vi "Main Draft LIEF Imager.vi"() -> ()   [LabVIEW 2016]
uses:
  Imager Editor Handler/Imager Handler.lvclass
  C:/Program Files (x86)/National Instruments/LabVIEW 2016/vi.lib/LIEF/Image Editor Handler/Image Editor Handler.lvclass
  Imager Editor Handler/Imager Handler.lvclass/Imager Handler.ctl
  Imager Editor Handler/Write Properties Pane.vi
  Imager Editor Handler/Write SystemPropertyChanged Event.vi
  <vilib>/LIEF/Image Editor Handler/Image Editor Handler.lvclass
  <vilib>/nisyscfg/nisyscfg.lvlib
panel:
  in  "Search":bool
  in  "Collapse":bool caption="Last"
  in  "2D Picture":picture
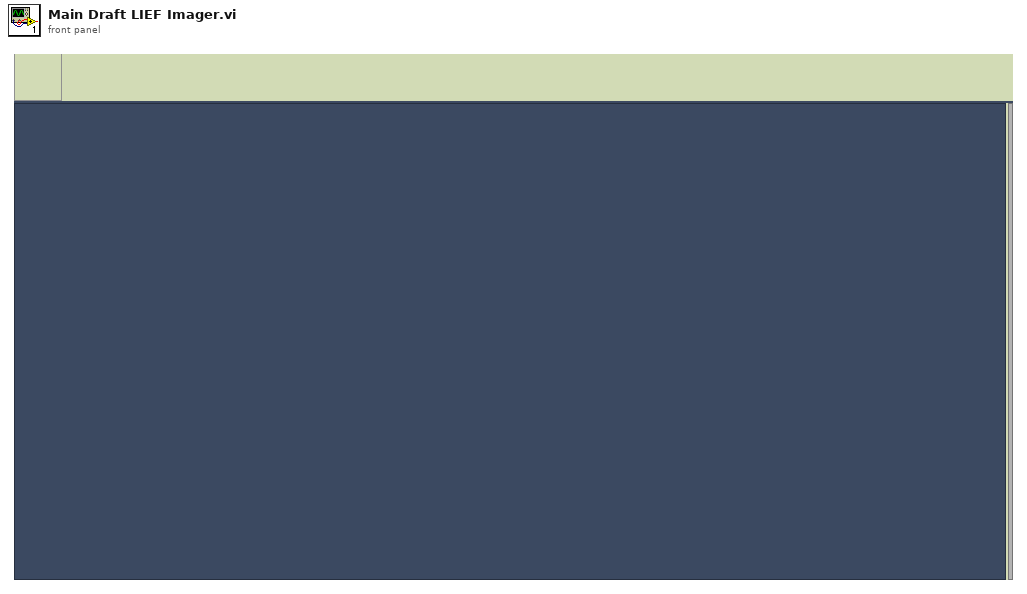
[diagram p1: front panel]
types:
  T1 = enum32{"invalid app kind", "Development System", "Run Time System", "Student Edition", "Embedded LabVIEW", "Evaluation", "Custom"}
  T2 = typedef "LVBoundsTypeDef.ctl" = cluster{"Width":u32, "Height":u32}
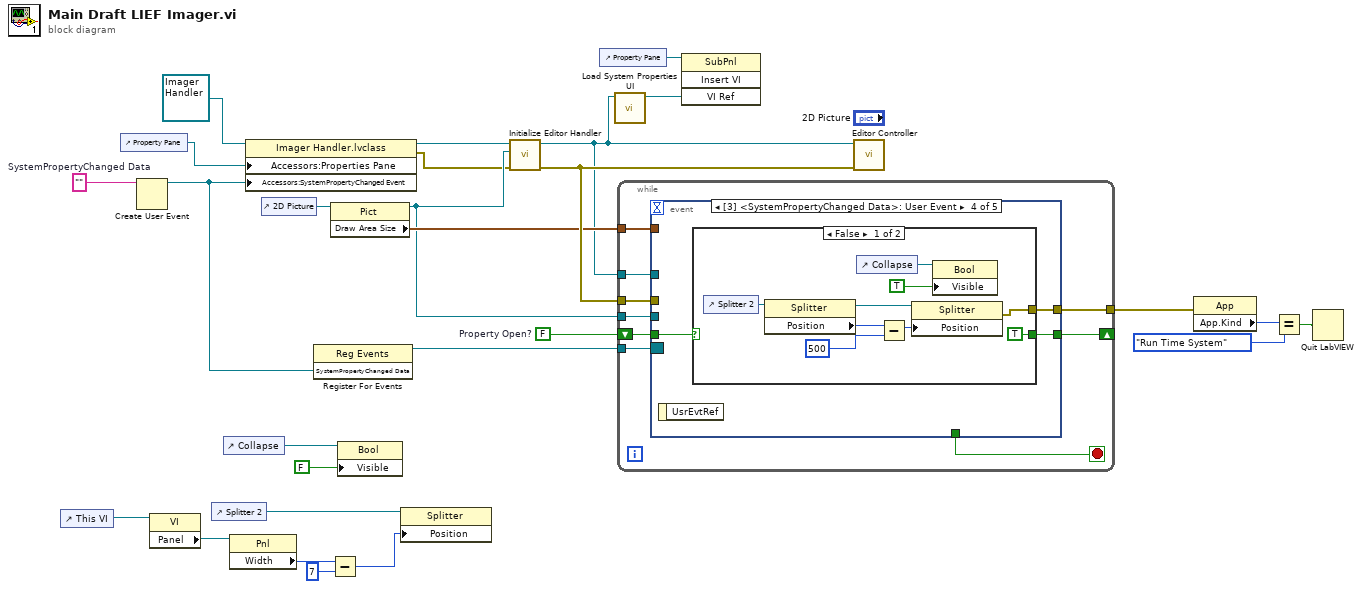
[diagram p0: block diagram]
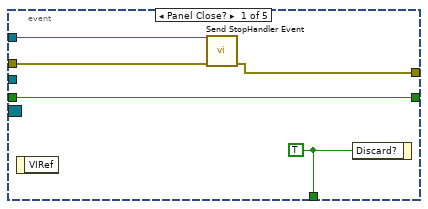
[diagram p2: hidden frame]
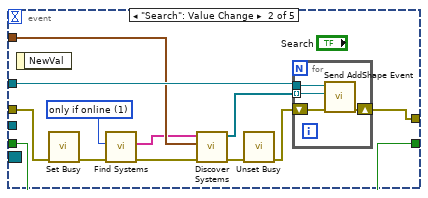
[diagram p3: hidden frame]
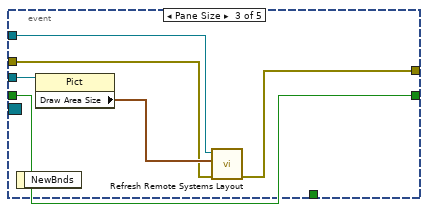
[diagram p4: hidden frame]
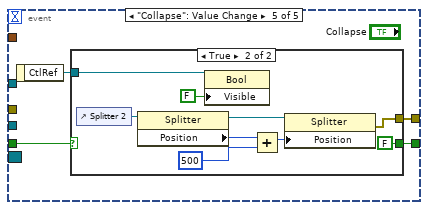
[diagram p6: hidden frame]
diagram:
  w15 = FALSE  # Property Open?
  w24 = ""  # SystemPropertyChanged Data
  n1 = control-ref of="This VI"() -> (w14:refnum<vi>)
  n2 = control-ref of="Property Pane"() -> (w18:refnum<vi>)
  n3 = Create User Event(user event datatype=w24) -> (user event=w20:refnum<user-event>)  [unwired: 1 in, 1 out]
  n4 = property class="VI"(reference=w14) -> ("Panel"=w13:refnum<vi>)  [unwired: 1 in, 2 out]
  n5 = control-ref of="Splitter 2"() -> (w12:refnum<vi>)
  n6 = control-ref of="Collapse"() -> (w17:refnum<vi>)
  n7 = property class="Pnl"(reference=w13) -> ("Width"=w11:u32)  [unwired: 1 in, 2 out]
  n8 = property class="Imager Handler.lvclass"(reference=refnum<class "Imager Handler.lvclass"> refnum ("Imager Handler.lvclass"), "Accessors:Properties Pane"=w18, "Accessors:SystemPropertyChanged Event"=w20) -> (reference out=w22:refnum<class "Imager Handler.lvclass">, error out=w5:errorcluster)  [unwired: 1 in]
  n9 = control-ref of="2D Picture"() -> (w27:refnum<vi>)
  n10 = register-events(w20) -> (reference out=w19:refnum<event-registration>)  [unwired: 2 in, 1 out]
  n11 = Subtract(x=w11, y=u32 7) -> (x-y=w9:u32)
  n12 = property class="Pict"(reference=w27) -> (reference out=w21:refnum<vi>, "Draw Area Size"=w25:T2)  [unwired: 1 in, 1 out]
  n13 = property class="Bool"(reference=w17, "Visible"=FALSE) -> ()  [unwired: 1 in, 2 out]
  n14 = property class="Splitter"(reference=w12, "Position"=w9) -> ()  [unwired: 1 in, 2 out]
  n15 = call <vilib>:"Initialize Editor Handler.vi"("error in (no error)"=w5, "PictureRef"=w21, "Editor Handler in"=w22) -> ("error out"=w26:errorcluster, "Editor Handler out"=w6:refnum<class "Imager Handler.lvclass">)  [unwired: 7 in]
  n16 = control-ref of="Property Pane"() -> (w8:refnum<vi>)
  n17 = call "Load System Properties UI.vi"("Editor Handler out"=w6) -> ("VI out"=w7:refnum<vi>)  [unwired: 9 in, 1 out]
  n18 = while {
    tunnel: w6 -> [w35]
    tunnel: w26 -> [w34]
    tunnel: w25 -> [w33]
    tunnel: w21 -> [w32]
    tunnel: w19 -> [w31]
    shift-right: [w29] -> _
    shift-left: w15 -> [w30]
    tunnel: [w28] -> w1
    stop <- w36 stop-if-true
    n19 = event shown="[3] <SystemPropertyChanged Data>: User Event" {
      selector: w31 -> [_ _ _ _ _]
      dyn-events: _ -> [_ _ _ _ _]
      timeout: _ -> [_ _ _ _ _]
      tunnel: [w41 _ _ _ _] -> w36
      tunnel: w35 -> [w40 w51 w59 _ _]
      tunnel: w34 -> [w39 w53 w61 _ _]
      tunnel: w33 -> [_ w50 _ _ _]
      tunnel: w32 -> [_ _ w63 _ _]
      tunnel: w30 -> [w38 w43 w60 w66 w79]
      tunnel: [w38 w43 w60 w65 w78] -> w29
      tunnel: [w37 w42 w58 w64 w77] -> w28
      event Panel Close? {
        w41 = TRUE ("Discard?")
        n20 = event-data() -> ()  [unwired: 1 in, 1 out]
        n21 = call <vilib>:"Send StopHandler Event.vi"("error in (no error)"=w39, "Editor Handler in"=w40) -> ("error out"=w37:errorcluster)  [unwired: 8 in, 1 out]
        n22 = event-data("Discard?"=w41) -> ()  [unwired: 1 in, 1 out]
      }
      event "Search": Value Change {
        w48 = u32 1 items=["none"=0, "only if online"=1, "all"=3] ("Include Cached Results (all)")
        n23 = event-data() -> ()  [unwired: 1 in, 1 out]
        n24 = call <vilib>:"Set Busy.vi"("error in (no error)"=w53) -> ("error out"=w47:errorcluster)  [unwired: 9 in, 1 out]
        n25 = call <vilib>:"Find Systems.vi"("error in (no error)"=w47, "Include Cached Results (all)"=w48) -> ("error out"=w46:errorcluster, "Detected Systems"=w45:string[])  [unwired: 7 in, 1 out]
        n26 = call "Discover Systems.vi"("error in (no error)"=w46, "Draw Area Size"=w50, "Detected Systems"=w45) -> ("error out"=w52:errorcluster, "RemoteSys Found"=w44:refnum<data-value>[])  [unwired: 5 in, 2 out]
        n27 = call <vilib>:"Unset Busy.vi"("error in (no error)"=w52) -> ("error out"=w49:errorcluster)  [unwired: 10 in]
        n28 = for {
          tunnel: w51 -> [w57]
          tunnel: w44 -> [w56] mode=indexing
          shift-right: [w54] -> w42
          shift-left: w49 -> [w55]
          n29 = call <vilib>:"Send AddShape Event.vi"("error in (no error)"=w55, "New Shape Reference"=w56, "Editor Handler in"=w57) -> ("error out"=w54:errorcluster)  [unwired: 7 in, 1 out]
        }
      }
      event Pane Size {
        n30 = event-data() -> ()  [unwired: 1 in, 1 out]
        n31 = property class="Pict"(reference=w63) -> ("Draw Area Size"=w62:T2)  [unwired: 1 in, 2 out]
        n32 = call "Refresh Remote Systems Layout.vi"("error in (no error)"=w61, "Draw Area Size"=w62, "Editor Handler in"=w59) -> ("error out"=w58:errorcluster)  [unwired: 8 in]
      }
      event User Event {
        n33 = event-data() -> ()  [unwired: 1 in, 1 out]
        n34 = case shown="False" w66 {
          selector: w66 -> [_ w76]
          tunnel: [TRUE ("Visible") w76] -> w65
          tunnel: [w67 _] -> w64
          frame False {
            n35 = control-ref of="Splitter 2"() -> (w75:refnum<vi>)
            n36 = property class="Splitter"(reference=w75) -> (reference out=w72:refnum<vi>, "Position"=w74:i32)  [unwired: 1 in, 1 out]
            n37 = control-ref of="Collapse"() -> (w70:refnum<vi>)
            n38 = Subtract(x=w74, y=500) -> (x-y=w71:i32)
            n39 = property class="Splitter"(reference=w72, "Position"=w71) -> (error out=w67:errorcluster)  [unwired: 1 in, 1 out]
            n40 = property class="Bool"(reference=w70, "Visible"=TRUE) -> ()  [unwired: 1 in, 2 out]
          }
          frame True {
          }
        }
      }
      event "Collapse": Value Change {
        n41 = event-data() -> ("CtlRef"=w80:refnum<vi>)  [unwired: 1 in]
        n42 = case shown="True" w79 {
          selector: w79 -> [w81 _]
          tunnel: w80 -> [_ w90]
          tunnel: [w81 FALSE ("Visible")] -> w78
          tunnel: [_ w82] -> w77
          frame False {
          }
          frame True {
            n43 = control-ref of="Splitter 2"() -> (w88:refnum<vi>)
            n44 = property class="Splitter"(reference=w88) -> (reference out=w85:refnum<vi>, "Position"=w87:i32)  [unwired: 1 in, 1 out]
            n45 = property class="Bool"(reference=w90, "Visible"=FALSE) -> ()  [unwired: 1 in, 2 out]
            n46 = Add(x=w87, y=500) -> (x+y=w84:i32)
            n47 = property class="Splitter"(reference=w85, "Position"=w84) -> (error out=w82:errorcluster)  [unwired: 1 in, 1 out]
          }
        }
      }
    }
  }
  n48 = invoke class="SubPnl" method="Insert VI"(reference=w8, "VI Ref"=w7) -> ()  [unwired: 2 in, 4 out]
  n49 = call <vilib>:"Editor Controller.vi"("error in (no error)"=w26, "Editor Handler in"=w6) -> ()  [unwired: 8 in, 2 out]
  n50 = property class="App"(error in=w1) -> ("App.Kind"=w4:T1)  [unwired: 1 in, 2 out]
  n51 = Equal?(x=w4, y=T1."Run Time System") -> (x = y?=w2:bool)
  n52 = Quit LabVIEW(quit? (T)=w2) -> ()
